vi "getTemperature.vi"(8 "error in (no error)":errorcluster, 10 "Reading Option (0: Latest)":i32, 11 "Electrometer in":refnum<class "Electrometer.lvclass">) -> (0 "error out":errorcluster, 1 "Temperature":string, 3 "Electrometer out":refnum<class "Electrometer.lvclass">)   [LabVIEW 2016, in "Electrometer.lvclass"]
uses:
  Electrometer.lvclass
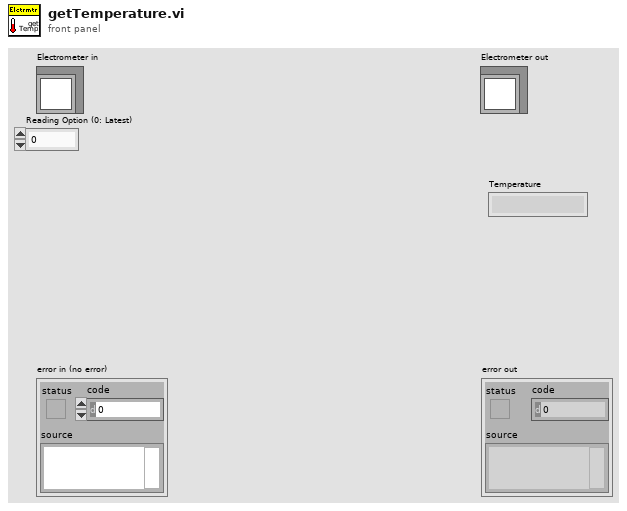
[diagram p1: front panel]
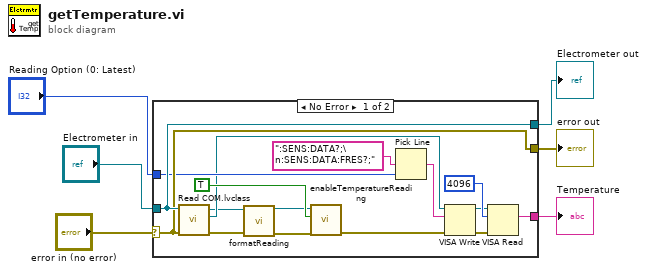
[diagram p0: block diagram]
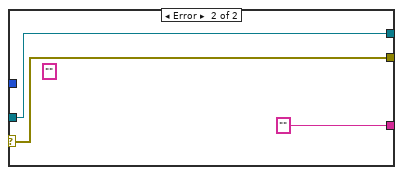
[diagram p2: hidden frame]
diagram:
  n1 = case shown="No Error" "error in (no error)" {
    selector: "error in (no error)" -> [w19 w25]
    tunnel: [w19 w25] -> w5
    tunnel: [w20 w24] -> w3
    tunnel: "Electrometer in" -> [w20 w24]
    tunnel: "Reading Option (0: Latest)" -> [w16 _]
    tunnel: [w14 "" ("read buffer")] -> w1
    frame No Error {
      n2 = call "Read COM.lvclass.vi"("error in (no error)"=w19, "Electrometer in"=w20) -> ("error out"=w9:errorcluster, "VISA"=w11:refnum<visa-resource-name>, "Electrometer out"=w10:refnum<class "Electrometer.lvclass">)  [unwired: 7 in]
      n3 = call "formatReading.vi"("error in (no error)"=w9, "Electrometer in"=w10) -> ("error out"=w8:errorcluster, "Electrometer out"=w7:refnum<class "Electrometer.lvclass">)  [unwired: 8 in]
      n4 = call "enableTemperatureReading.vi"("error in (no error)"=w8, "Enable Temperature (T: Enable)"=TRUE, "Electrometer in"=w7) -> ("error out"=w13:errorcluster)  [unwired: 7 in, 1 out]
      n5 = Pick Line(multi-line string=":SENS:DATA?;\n:SENS:DATA:FRES?;", line index=w16) -> (output string=w17:string)  [unwired: 1 in]
      n6 = VISA Write(VISA resource name=w11, write buffer=w17, error in (no error)=w13) -> (VISA resource name out=w21:refnum<visa-resource-name>, error out=w18:errorcluster)  [unwired: 1 out]
      n7 = VISA Read(VISA resource name=w21, byte count=u32 4096, error in (no error)=w18) -> (read buffer=w14:string)  [unwired: 3 out]
    }
    frame Error {
      (unwired) "" ("read buffer")
    }
  }
  "error out" <- w5
  "Electrometer out" <- w3
  "Temperature" <- w1
